vi "getName.vi"(8 "error in (no error)":errorcluster, 11 "vehicleGeneric in":refnum<class "vehicleGeneric.lvclass">) -> (0 "error out":errorcluster, 2 "name":string, 3 "vehicleGeneric out":refnum<class "vehicleGeneric.lvclass">)   [LabVIEW 2011, in "vehicleGeneric.lvclass"]
uses:
  vehicleGeneric.lvclass
  vehicleGeneric.lvclass/vehicleGeneric.ctl
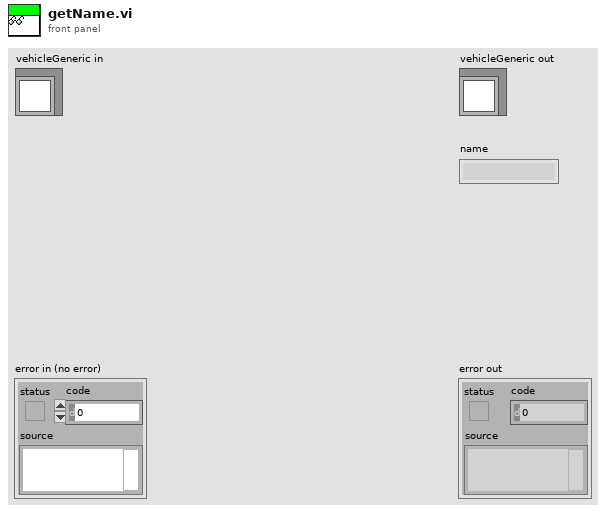
[diagram p1: front panel]
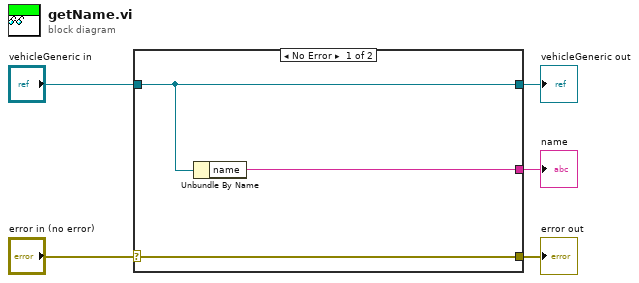
[diagram p0: block diagram]
diagram:
  n1 = case shown="No Error" "error in (no error)" {
    selector: "error in (no error)" -> [w8 w9]
    tunnel: [w8 w9] -> w4
    tunnel: [w7 w10] -> w2
    tunnel: "vehicleGeneric in" -> [w7 w10]
    tunnel: [w6 _] -> w1
    frame No Error {
      n2 = Unbundle By Name(w7) -> ("name"=w6:string)
    }
    frame Error {
    }
  }
  "error out" <- w4
  "vehicleGeneric out" <- w2
  "name" <- w1
